vi "Broacast de Prueba.vi"(8 "error in (no error)":errorcluster, 10 "Valor de Prueba":dbl) -> (0 "error out":errorcluster)   [LabVIEW 2020, in "Graficas.lvlib"]
doc: "_____\nCreated using Delacor QMH Event Scripter 5.0.0.112."
uses:
  Graficas.lvlib
  Broacast de Prueba Argument--cluster.ctl
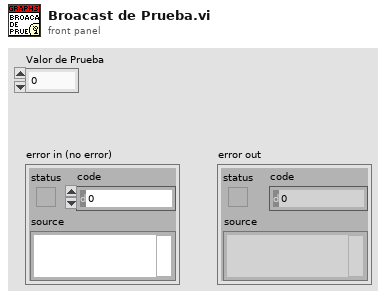
[diagram p1: front panel]
types:
  T1 = typedef "Graficas.lvlib/Broacast de Prueba Argument--cluster.ctl" = cluster{"Valor de Prueba":dbl}
  T2 = typedef "Graficas.lvlib/Broadcast Events--cluster.ctl" = cluster{"Module Did Init":refnum<user-event>, "Status Updated":refnum<user-event>, "Error Reported":refnum<user-event>, "Module Did Stop":refnum<user-event>, "Update Module Execution Status":refnum<user-event>, "Broacast de Prueba":refnum<user-event>}
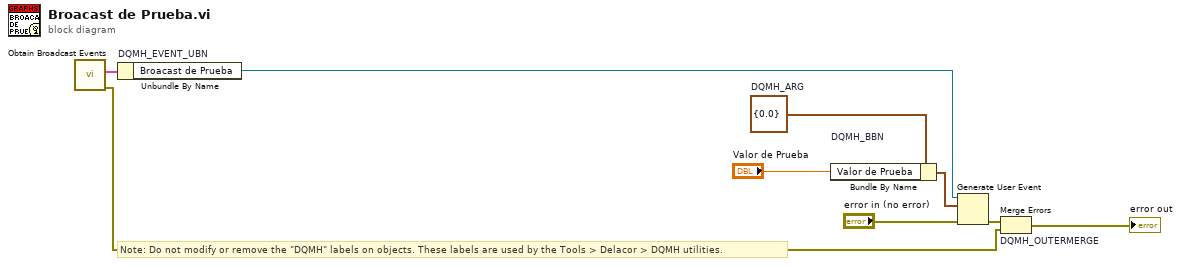
[diagram p0: block diagram]
diagram:
  w4 = T1 {"Valor de Prueba"=0.0}  # DQMH_ARG
  # "Note: Do not modify or remove the \"DQMH\" labels on objects. These labels are used by the Tools > Delacor > DQMH utilities."
  n1 = call "Obtain Broadcast Events.vi"() -> ("error out"=w2:errorcluster, "Graficas Broadcast Events"=w1:T2)  [unwired: 10 in]
  n2 = Unbundle By Name "DQMH_EVENT_UBN"(w1) -> ("Broacast de Prueba"=w6:refnum<user-event>)
  n3 = Bundle By Name "DQMH_BBN"(cluster=w4, "Valor de Prueba"="Valor de Prueba") -> (w7:T1)
  n4 = Generate User Event(user event=w6, event data cluster=w7, error in="error in (no error)") -> (error out=w5:errorcluster)  [unwired: 1 in, 1 out]
  n5 = Merge Errors "DQMH_OUTERMERGE"(w5, w2) -> (→"error out":errorcluster)
